vi "Cluster---Array.vi"(2 "Array (A) in":dbl[][](array[numeric])=[[1.0, 0.0, 0.0, 5.0], [0.0, 3.0, 0.0, 2.0], [0.0, 0.0, 4.0, 3.0], [0.0, 0.0, 0.0, 1.0]] format="%.2f", 3 "A":T1={"nx"=1.0, "ny"=0.0, "nz"=0.0, "nw"=0.0, "ox"=0.0, "oy"=3.0, "oz"=0.0, "ow"=0.0, "ax"=0.0, "ay"=0.0, "az"=4.0, "aw"=0.0, "Px"=5.0, "Py"=2.0, "Pz"=3.0, "Pw"=1.0} {"Pw" format="%.2f"; "Pz" format="%.2f"; "Py" format="%.2f"; "Px" format="%.2f"; "aw" format="%.2f"; "az" format="%.2f"; "ay" format="%.2f"; "ax" format="%.2f"; "ow" format="%.2f"; "nw" format="%.2f"; "oz" format="%.2f"; "oy" format="%.2f"; "ox" format="%.2f"; "nz" format="%.2f"; "ny" format="%.2f"; "nx" format="%.2f"}) -> (0 "A":T1={"nx"=1.0, "ny"=0.0, "nz"=0.0, "nw"=0.0, "ox"=0.0, "oy"=3.0, "oz"=0.0, "ow"=0.0, "ax"=0.0, "ay"=0.0, "az"=4.0, "aw"=0.0, "Px"=5.0, "Py"=2.0, "Pz"=3.0, "Pw"=1.0} {"Pw" format="%.2f"; "Pz" format="%.2f"; "Py" format="%.2f"; "Px" format="%.2f"; "aw" format="%.2f"; "az" format="%.2f"; "ay" format="%.2f"; "ax" format="%.2f"; "ow" format="%.2f"; "nw" format="%.2f"; "oz" format="%.2f"; "oy" format="%.2f"; "ox" format="%.2f"; "nz" format="%.2f"; "ny" format="%.2f"; "nx" format="%.2f"}, 1 "Array (A)":dbl[][](array[numeric])=[[1.0, 0.0, 0.0, 5.0], [0.0, 3.0, 0.0, 2.0], [0.0, 0.0, 4.0, 3.0], [0.0, 0.0, 0.0, 1.0]] format="%.2f")   [LabVIEW 2010]
uses:
  ReferenceFrame.ctl
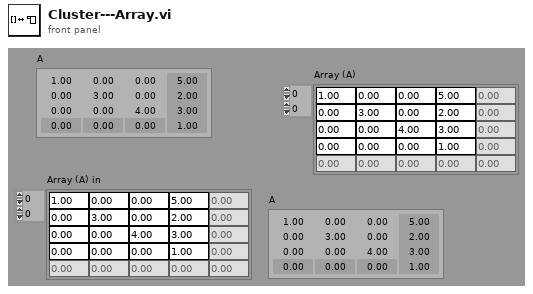
[diagram p1: front panel]
types:
  T1 = typedef "ReferenceFrame.ctl" = cluster{"nx":dbl, "ny":dbl, "nz":dbl, "nw":dbl, "ox":dbl, "oy":dbl, "oz":dbl, "ow":dbl, "ax":dbl, "ay":dbl, "az":dbl, "aw":dbl, "Px":dbl, "Py":dbl, "Pz":dbl, "Pw":dbl}
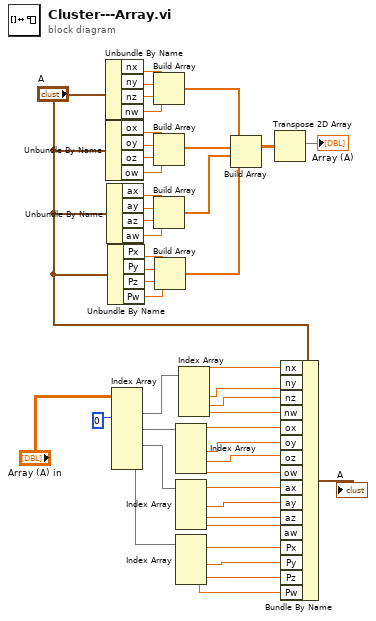
[diagram p0: block diagram]
diagram:
  n1 = Unbundle By Name("A") -> ("nx"=w38:dbl, "ny"=w39:dbl, "nz"=w40:dbl, "nw"=w37:dbl)
  n2 = Unbundle By Name("A") -> ("ox"=w43:dbl, "oy"=w42:dbl, "oz"=w41:dbl, "ow"=w35:dbl)
  n3 = Unbundle By Name("A") -> ("ax"=w44:dbl, "ay"=w45:dbl, "az"=w46:dbl, "aw"=w36:dbl)
  n4 = Unbundle By Name("A") -> ("Px"=w34:dbl, "Py"=w33:dbl, "Pz"=w32:dbl, "Pw"=w31:dbl)
  n5 = Index Array(array="Array (A) in", index (col) #1=0) -> (element #1=w22:dbl[], element #2=w16:dbl[], element #3=w11:dbl[], element #4=w6:dbl[])  [unwired: 7 in]
  n6 = Build Array(w38, w39, w40, w37) -> (w30:dbl[])
  n7 = Build Array(w43, w42, w41, w35) -> (w29:dbl[])
  n8 = Build Array(w44, w45, w46, w36) -> (w28:dbl[])
  n9 = Build Array(w34, w33, w32, w31) -> (w27:dbl[])
  n10 = Index Array(array=w16) -> (element #1=w15:dbl, element #2=w14:dbl, element #3=w13:dbl, element #4=w12:dbl)  [unwired: 4 in]
  n11 = Index Array(array=w11) -> (element #1=w10:dbl, element #2=w9:dbl, element #3=w8:dbl, element #4=w7:dbl)  [unwired: 4 in]
  n12 = Index Array(array=w6) -> (element #1=w5:dbl, element #2=w4:dbl, element #3=w3:dbl, element #4=w2:dbl)  [unwired: 4 in]
  n13 = Index Array(array=w22) -> (element #1=w20:dbl, element #2=w19:dbl, element #3=w18:dbl, element #4=w17:dbl)  [unwired: 4 in]
  n14 = Build Array(w30, w29, w28, w27) -> (w26:dbl[][])
  n15 = Transpose 2D Array(2D array=w26) -> (transposed array=→"Array (A)":dbl[][])
  n16 = Bundle By Name(cluster="A", "nx"=w20, "ny"=w19, "nz"=w18, "nw"=w17, "ox"=w15, "oy"=w14, "oz"=w13, "ow"=w12, "ax"=w10, "ay"=w9, "az"=w8, "aw"=w7, "Px"=w5, "Py"=w4, "Pz"=w3, "Pw"=w2) -> (→"A":T1)
